vi "UpDataResult.vi"(8 "error in (no error)":errorcluster, 9 "Time":dbl, 10 "UpDataResult":T1={"Slot"=-1, "Result"="EXIT", "Value"="", "Limit"={"High"="", "Low"=""}, "Type"="", "StepName"="", "Normal"="", "Unit"=""}, 11 "UnitTestEngine in":refnum<class "UnitTestEngine.lvclass">) -> (0 "error out":errorcluster, 3 "UnitTestEngine out":refnum<class "UnitTestEngine.lvclass">)   [LabVIEW 2019, in "UnitTestEngine.lvlib" / "UnitTestEngine.lvclass"]
uses:
  UnitTestEngine.lvclass
  C:/Program Files (x86)/National Instruments/LabVIEW 2019/vi.lib/NI/Event Source Actor/Event Source/Event Source/Event Source.lvclass
  <vilib>/Utility/miscctls.llb/LVRowAndColumnUnsignedTypeDef.ctl
  <vilib>/Utility/miscctls.llb/LVRowAndColumnTypeDef.ctl
  TestEngine/TestEngine/TestDetailedResult.lvclass
  C:/Program Files (x86)/National Instruments/LabVIEW 2019/vi.lib/NI/Event Source Actor/Event Source/Event/Event.lvclass
  <vilib>/NI/Event Source Actor/Event Source/Event/Event.lvclass/Event.ctl
  UnitTestEngine.lvclass/UnitTestEngine.ctl
  <vilib>/NI/Event Source Actor/Event Source/Event/Event.lvclass
  <vilib>/NI/Event Source Actor/Event Source/Event Source/Event Source.lvclass
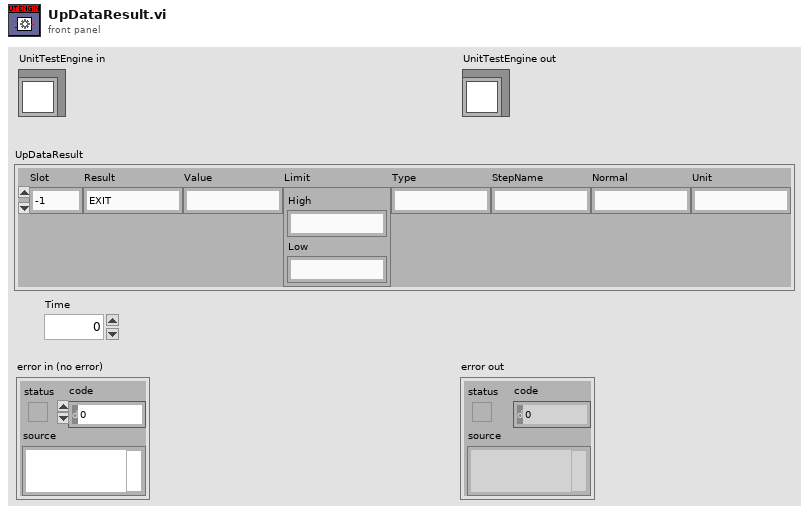
[diagram p1: front panel]
types:
  T1 = cluster{"Slot":i32, "Result":string, "Value":string, "Limit":cluster{"High":string, "Low":string}, "Type":string, "StepName":string, "Normal":string, "Unit":string}
  T2 = typedef "LVRowAndColumnTypeDef.ctl" = cluster{"Row":i32, "Column":i32}
  T3 = typedef "LVRowAndColumnUnsignedTypeDef.ctl" = cluster{"Row":u32, "Column":u32}
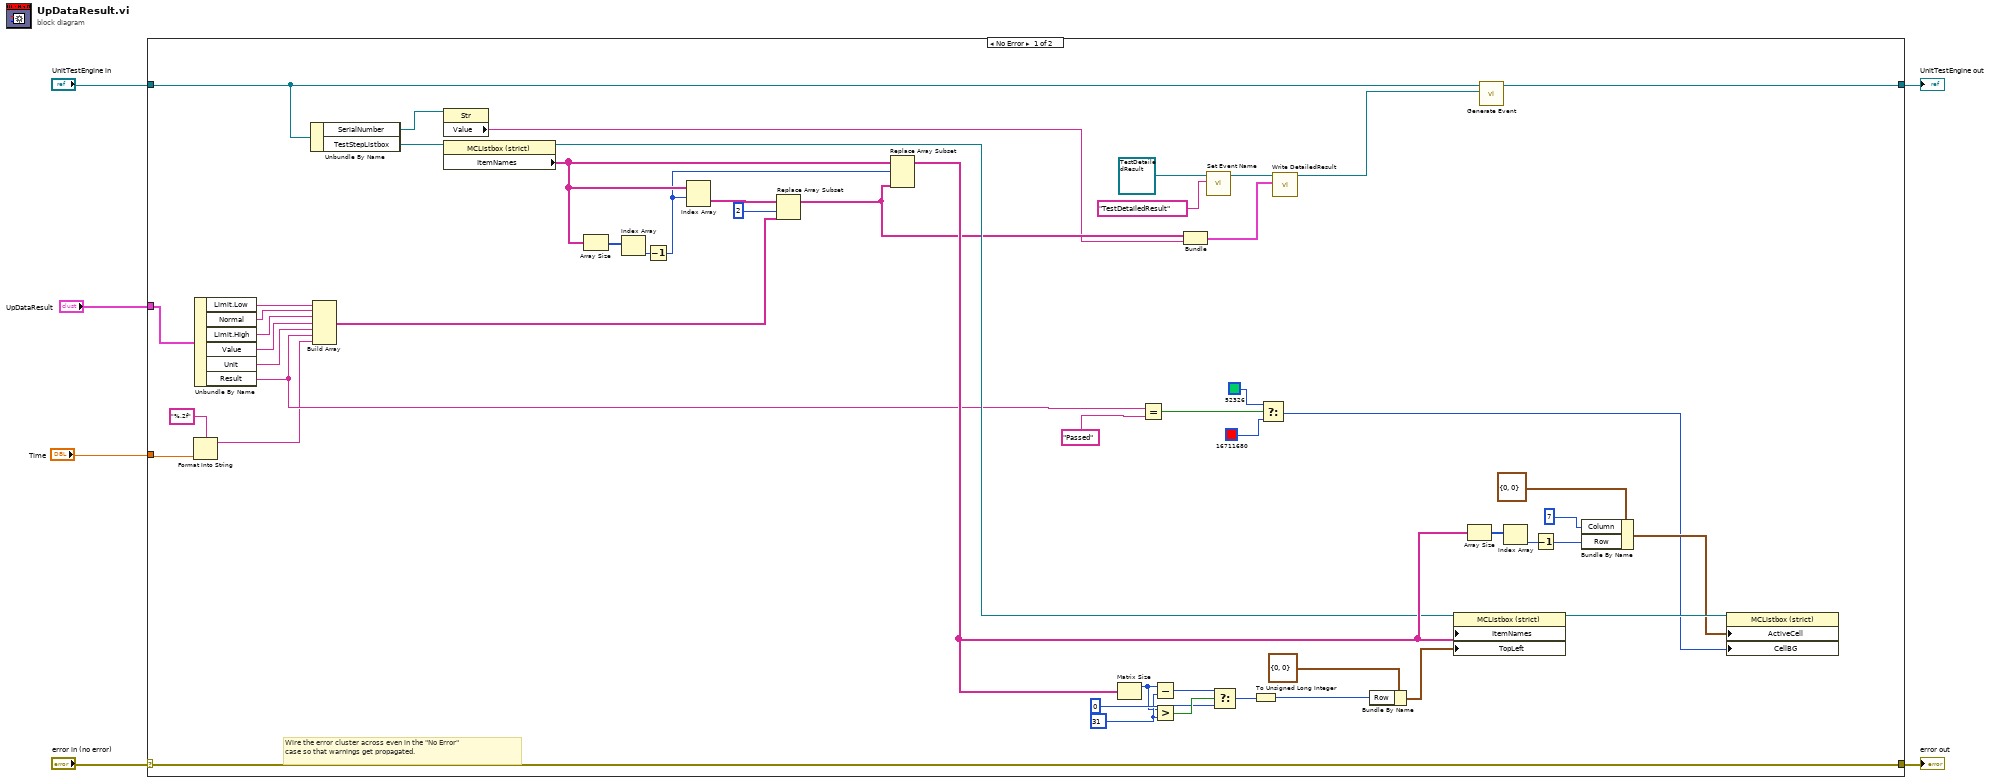
[diagram p0: block diagram]
diagram:
  n1 = case shown="No Error" "error in (no error)" {
    selector: "error in (no error)" -> [w58 w60]
    tunnel: [w58 w60] -> w5
    tunnel: [w8 w59] -> w3
    tunnel: "UnitTestEngine in" -> [w9 w59]
    tunnel: "UpDataResult" -> [w57 _]
    tunnel: "Time" -> [w19 _]
    frame No Error {
      w35 = 31
      # "Wire the error cluster across even in the \"No Error\"\ncase so that warnings get propagated."
      n2 = Format Into String(format string="%.2f", w19) -> (resulting string=w17:string)  [unwired: 2 in, 1 out]
      n3 = Unbundle By Name(w57) -> ("Limit.Low"=w51:string, "Normal"=w50:string, "Limit.High"=w49:string, "Value"=w48:string, "Unit"=w47:string, "Result"=w21:string)
      n4 = Unbundle By Name(w9) -> ("SerialNumber"=w11:refnum<vi>, "TestStepListbox"=w56:refnum<vi>)
      n5 = Build Array(w51, w50, w49, w48, w47, w21, w17) -> (w46:string[])
      n6 = property class="Str"(reference=w11) -> ("Value"=w10:string)  [unwired: 1 in, 2 out]
      n7 = property class="MCListbox (strict)"(reference=w56) -> (reference out=w27:refnum<vi>, "ItemNames"=w45:string[][])  [unwired: 1 in, 1 out]
      n8 = Array Size(array=w45) -> (size(s)=w55:i32[])
      n9 = Index Array(array=w55) -> (element=w54:i32)  [unwired: 1 in]
      n10 = Decrement(x=w54) -> (x-1=w44:i32)
      n11 = Index Array(array=w45, index (row)=w44) -> (element=w53:string[])  [unwired: 1 in]
      n12 = Replace Array Subset(array=w53, new element=w46, index=2) -> (w12:string[])
      n13 = Replace Array Subset(array=w45, new element=w12, index (row)=w44) -> (w28:string[][])  [unwired: 1 in]
      n14 = Matrix Size(0:w28) -> (1:w34:i32)  [unwired: 1 out]
      n15 = Equal?(x=w21, y="Passed") -> (x = y?=w30:bool)
      n16 = Subtract(x=w34, y=w35) -> (x-y=w38:i32)
      n17 = Greater?(x=w34, y=w35) -> (0:w40:bool)
      n18 = Bundle("ItemNames"=w12, "Value"=w10) -> (w13:cluster{"ItemNames":string[], "Value":string})  [unwired: 1 in]
      n19 = call <vilib>:"Set Event Name.vi"("Name (Generic)"="TestDetailedResult", "Event In"=refnum<class "TestDetailedResult.lvclass"> refnum ("TestEngine.lvlib:TestDetailedResult.lvclass")) -> ("Event Out"=w14:refnum<class "TestDetailedResult.lvclass">)  [unwired: 9 in]
      n20 = Select(t=w38, s=w40, f=0) -> (s? t:f=w37:i32)
      n21 = To Unsigned Long Integer(number=w37) -> (unsigned 32bit integer=w41:u32)
      n22 = Select(t=u32 52326 ("Text.Text Colors:Text Color"), s=w30, f=u32 16711680 ("Text.Text Colors:Text Color")) -> (s? t:f=w29:u32)
      n23 = call-dynamic "Write DetailedResult.vi"("DetailedResult"=w13, "TestDetailedResult in"=w14) -> ("TestDetailedResult out"=w7:refnum<class "TestDetailedResult.lvclass">)  [unwired: 8 in, 1 out]
      n24 = Bundle By Name(cluster=T3 {"Row"=0, "Column"=0} ("Top Left Visible Cell"), "Row"=w41) -> (w33:T3)
      n25 = property class="MCListbox (strict)"(reference=w27, "ItemNames"=w28, "TopLeft"=w33) -> (reference out=w43:refnum<vi>)  [unwired: 1 in, 1 out]
      n26 = Array Size(array=w28) -> (size(s)=w24:i32[])
      n27 = call <vilib>:"Generate Event.vi"("Event"=w7, "Event Source In"=w9) -> ("Event Source Out"=w8:refnum<class "UnitTestEngine.lvclass">)  [unwired: 8 in, 1 out]
      n28 = Index Array(array=w24) -> (element=w23:i32)  [unwired: 1 in]
      n29 = Decrement(x=w23) -> (x-1=w22:i32)
      n30 = Bundle By Name(cluster=T2 {"Row"=0, "Column"=0} ("Active Cell:Active Cell"), "Column"=7, "Row"=w22) -> (w42:T2)
      n31 = property class="MCListbox (strict)"(reference=w43, "ActiveCell"=w42, "CellBG"=w29) -> ()  [unwired: 1 in, 2 out]
    }
    frame Error {
    }
  }
  "error out" <- w5
  "UnitTestEngine out" <- w3
